vi "cogs.vi"() -> ()   [LabVIEW 2015]
panel:
  out "element":T1
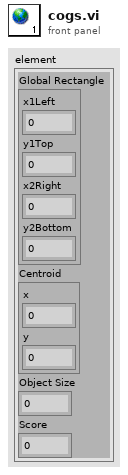
[diagram p1: front panel]
types:
  T1 = cluster{"Global Rectangle":cluster{"x1Left":i32, "y1Top":i32, "x2Right":i32, "y2Bottom":i32}, "Centroid":cluster{"x":sgl, "y":sgl}, "Object Size":u32, "Score":dbl}
diagram:
